vi "DAQmx Voltage Task.vi"() -> ()   [LabVIEW 2021]
uses:
  <vilib>/DAQmx/read.llb/DAQmx Read (Analog 1D DBL NChan 1Samp).vi
  <vilib>/DAQmx/miscellaneous.llb/DAQmx Fill In Error Info.vi
panel:
  out "Waveform Chart":T1(graph)
  in  "stop":bool
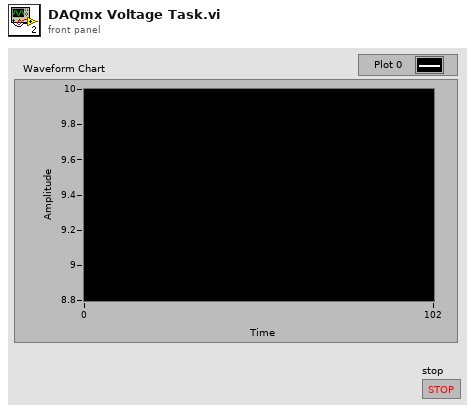
[diagram p1: front panel]
types:
  T1 = cluster{"data[0]":dbl, "data[1]":dbl, "data[2]":dbl, "data[3]":dbl}
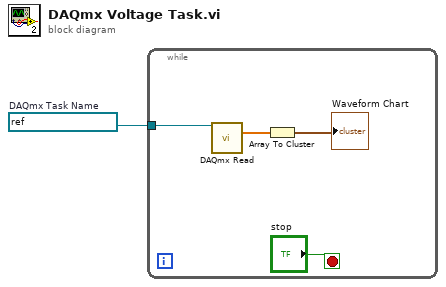
[diagram p0: block diagram]
diagram:
  w1 = refnum<k21> "MyVoltageTask"  # DAQmx Task Name
  n1 = while {
    tunnel: w1 -> [w5]
    stop <- "stop" stop-if-true
    n2 = call-poly <vilib>:"DAQmx Read.vi"("task/channels in"=w5) -> ("data"=w3:dbl[])  [unwired: 12 in, 2 out]
    n3 = Array To Cluster(array=w3) -> (cluster=→"Waveform Chart":T1)
  }
